vi "Incomplete Gamma Function.vi"(10 "a":dbl=inf format="%.2f", 11 "x":dbl format="%.2f") -> (3 "g(x, a)":dbl format="%.2f")   [LabVIEW 2020, in "NI_Gmath.lvlib"]
doc: "Evaluates the gamma function and regularized incomplete gamma function. You must manually select the polymorphic instance you want to use."
uses:
  NI_Gmath.lvlib
  <resource>/lvanlys.dll
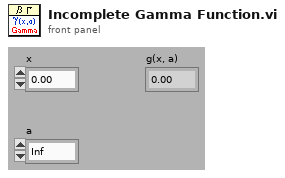
[diagram p1: front panel]
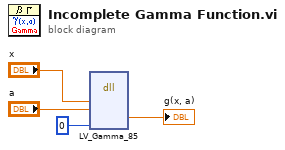
[diagram p0: block diagram]
diagram:
  n1 = dll-call lib="C:/Program Files (x86)/National Instruments/LabVIEW 2020/resource/lvanlys.*" fn="LV_Gamma_85"("x"="x", "a"="a", "funcType"=0) -> ("Gamma(x, a)"=→"g(x, a)":dbl)  [unwired: 8 in, 2 out]
